vi "SentinelController v35 good v11.vi"() -> ()   [LabVIEW 2011] (continued)
                                tunnel: w568 -> [w597]
                                shift-right: [w590] -> w555
                                shift-left: 0 -> [w589]
                                shift-right: [w586] -> w556
                                shift-left: 0 -> [w584]
                                i -> [w587]
                                n2144 = Increment(x=w584) -> (x+1=w585:i32)
                                n2145 = Increment(x=w589) -> (x+1=w588:i32)
                                n2146 = Increment(x=w587) -> (x+1=w605:i32)
                                n2147 = String Subset(string=w597, offset (0)=w587, length (rest)=1 ("length (rest)")) -> (substring=w593:string)
                                n2148 = Multiply(x=3, y=w605) -> (x*y=w599:i32)
                                n2149 = Equal?(x=w593, y="1") -> (x = y?=w591:bool)
                                n2150 = Decrement(x=w599) -> (x-1=w598:i32)
                                n2151 = Select(t=w588, s=w591, f=w589) -> (s? t:f=w590:i32)
                                n2152 = Index Array(array=w606, index=w598) -> (element=w603:string)
                                n2153 = Decimal String To Number(string=w603, offset=0) -> (number=w601:i32)  [unwired: 1 in, 1 out]
                                n2154 = Equal?(x=w601, y=1) -> (x = y?=w594:bool)
                                n2155 = And(x=w594, y=w591) -> (x .and. y?=w595:bool)
                                n2156 = Select(t=w585, s=w595, f=w584) -> (s? t:f=w586:i32)
                                }
                                n2157 = case shown="True" w572 {
                                frame False {
                                }
                                frame True {
                                n2158 = One Button Dialog(message="Warning:\nH1 Parallelism Mismatch!\nEither allow this from the system configuration tab\nor change the parallelism on H2. This message will\ncontinue until the problem is corrected.") -> ()  [unwired: 1 in, 1 out]
                                }
                                }
                                n2159 = local read "H1 Device Count"() -> (w564:u32)
                                n2160 = local read "H1 Good Units"() -> (w565:u32)
                                n2161 = Add(x=w565, y=w556) -> (x+y=w566:u32)
                                n2162 = Add(x=w564, y=w555) -> (x+y=w563:u32)
                                n2163 = local write "H1 Good Units"(w566) -> ()
                                n2164 = local write "H1 Device Count"(w563) -> ()
                                }
                                frame #4 {
                                n2165 = local read "H1 Device Count"() -> (w612:u32)
                                n2166 = Divide(x=w608, y=w607) -> (x/y=w609:dbl)
                                n2167 = local read "H1 Good Units"() -> (w613:u32)
                                n2168 = Multiply(x=w609, y=100.0) -> (x*y=w611:dbl)
                                n2169 = Divide(x=w613, y=w612) -> (x/y=w616:dbl)
                                n2170 = local write "H1 cycle yield hid"(w611) -> ()
                                n2171 = Multiply(x=w616, y=100.0) -> (x*y=w614:dbl)
                                n2172 = local write "H1 lot yield mon"(w614) -> ()
                                }
                                frame #5 {
                                n2173 = local read "H1 online"() -> (w617:bool)
                                n2174 = local read "POWER"() -> (w618:bool)
                                n2175 = Compound Arithmetic op=AND(w617, w618) -> (w619:bool)
                                n2176 = case shown="True" w619 {
                                frame False {
                                n2177 = local write "MT99XX tester states H1 hid"(SC_MT99XX_tester_states."closing bus" ("SC virtual tester states")) -> ()
                                }
                                frame True {
                                n2178 = local write "MT99XX tester states H1 hid"(SC_MT99XX_tester_states."polling *SITES?" ("SC virtual tester states")) -> ()
                                }
                                }
                                }
                                }
                                }
                                frame "closing bus" {
                                n2179 = local read "GPIB bus 1 traffic"() -> (w626:string)
                                n2180 = local write "Exit SC tester H1 StMach hid"(TRUE ("Exit H1 state machine hid")) -> ()
                                n2181 = local read "VISA bus 1 resource name out hid"() -> (w630:refnum<visa-resource-name>)
                                n2182 = local read "VISA bus 1 error out hid"() -> (w629:errorcluster)
                                n2183 = Concatenate Strings(w626, "\r\n", "Bus 1: closing " ("string")) -> (w624:string)
                                n2184 = local write "GPIB bus 1 traffic"(w624) -> ()
                                n2185 = VISA Close(VISA resource name=w630, error in (no error)=w629) -> (error out=w628:errorcluster)
                                n2186 = Unbundle By Name(w628) -> ("status"=w627:bool)
                                n2187 = local write "VISA bus 1 close error"(w627) -> ()
                                }
                              }
                            }
                            frame #1 {
                              n2188 = local read "Slow for  Diagnostics"() -> (w631:bool)
                              n2189 = case shown="False" w631 {
                                frame False {
                                }
                                frame True {
                                n2190 = local read "GPIB wait time (ms)"() -> (w632:u32)
                                n2191 = Wait (ms)(milliseconds to wait=w632) -> ()  [unwired: 1 out]
                                }
                              }
                            }
                          }
                        }
                        frame "Seiko-Epson NS6040" {
                          n2192 = local write "NS6040 tester states H1 hid"(SC_NS6040_tester_states."initializing bus" ("NS6040 tester states H1 hid")) -> ()
                          n2193 = while {
                            stop <- w634 stop-if-true
                            n2194 = flat-sequence {
                              frame #0 {
                                n2195 = local read "NS6040 tester states H1 hid"() -> (w635:T4)
                                n2196 = case shown="\"testing\"" w635 {
                                frame "initializing bus", Default {
                                n2197 = flat-sequence {
                                frame #0 {
                                # "bus 1"
                                n2198 = local read "GPIB wait timeout hid"() -> (w639:u32)
                                n2199 = local read "SentCtrl talks to handler 1 at"() -> (w640:refnum<visa-resource-name>)
                                n2200 = local read "GPIB wait timeout hid"() -> (w638:u32)
                                n2201 = VISA Open(timeout (0)=w639, VISA resource name=w640) -> (VISA resource name=w637:refnum<visa-resource-name>, error out=w642:errorcluster)  [unwired: 3 in]
                                n2202 = property class="GPIB Instr"(reference=w637, error in=w642, "Timeout"=w638) -> (error out=w636:errorcluster)  [unwired: 1 out]
                                n2203 = local write "VISA bus 1 resource name out hid"(w637) -> ()
                                n2204 = Unbundle By Name(w636) -> ("status"=w641:bool)
                                n2205 = local write "VISA bus 1 open error"(w641) -> ()
                                n2206 = local write "VISA bus 1 error out hid"(w636) -> ()
                                }
                                frame #1 {
                                n2207 = local write "Exit SC tester H1 StMach hid"(FALSE ("Exit H1 state machine hid")) -> ()
                                n2208 = Concatenate Strings("Bus 1 initializing" ("string"), "\r\n") -> (w645:string)
                                n2209 = local write "GPIB bus 1 traffic"(w645) -> ()
                                }
                                frame #2 {
                                n2210 = local write "NS6040 tester states H1 hid"(SC_NS6040_tester_states."serial polling handler" ("NS6040 tester states H1 hid")) -> ()
                                }
                                }
                                }
                                frame "sending *IDN?" {
                                n2211 = flat-sequence {
                                tunnel: [w657] -> w650
                                tunnel: [w656] -> w649
                                tunnel: w650 -> [w671]
                                tunnel: w649 -> [w670]
                                tunnel: [w661] -> w648
                                tunnel: w648 -> [w672]
                                frame #0 {
                                w651 = "*IDN?\n"
                                # "It was discovered that his state is not initialized in application"
                                n2212 = local read "VISA bus 1 resource name out hid"() -> (w660:refnum<visa-resource-name>)
                                n2213 = local read "GPIB bus 1 traffic"() -> (w655:string)
                                n2214 = local read "VISA bus 1 error out hid"() -> (w659:errorcluster)
                                n2215 = Concatenate Strings(w655, "\r\n", "Bus 1 write: " ("string"), w651) -> (w653:string)
                                n2216 = VISA Write(VISA resource name=w660, write buffer=w651, error in (no error)=w659) -> (VISA resource name out=w657:refnum<visa-resource-name>, error out=w656:errorcluster)  [unwired: 1 out]
                                n2217 = Unbundle By Name(w656) -> ("status"=w658:bool)
                                n2218 = local write "GPIB bus 1 traffic"(w653) -> ()
                                n2219 = local write "GPIB bus 1 write error"(w658) -> ()
                                }
                                frame #1 {
                                n2220 = local read "GPIB bus 1 traffic"() -> (w663:string)
                                n2221 = VISA Read(VISA resource name=w671, byte count=u32 256, error in (no error)=w670) -> (VISA resource name out=w668:refnum<visa-resource-name>, read buffer=w662:string, error out=w667:errorcluster)  [unwired: 1 out]
                                n2222 = local write "VISA bus 1 resource name out hid"(w668) -> ()
                                n2223 = Unbundle By Name(w667) -> ("status"=w661:bool)
                                n2224 = local write "H1 response to *IDN? hid"(w662) -> ()
                                n2225 = local write "GPIB bus 1 read error"(w661) -> ()
                                n2226 = Concatenate Strings(w663, "\r\n", "Bus 1 read: " ("string"), w662) -> (w665:string)
                                n2227 = local write "GPIB bus 1 traffic"(w665) -> ()
                                }
                                frame #2 {
                                n2228 = case shown="False" w672 {
                                frame False {
                                n2229 = local write "NS6040 tester states H1 hid"(SC_NS6040_tester_states."serial polling handler" ("NS6040 tester states H1 hid")) -> ()
                                }
                                frame True {
                                n2230 = flat-sequence {
                                frame #0 {
                                n2231 = while {
                                stop <- w675 stop-if-true
                                n2232 = One Button Dialog(message="Warning:\nVirtual tester does not get a response\nto *IDN? from handler 1.\nCheck GPIB cable and that  handler 1 \nis running and ready to issue a start of test\nby responding with sites ready.", button name ("OK")="Dismiss and retry") -> (true=w675:bool)
                                n2233 = Wait (ms)(milliseconds to wait=u32 100) -> ()  [unwired: 1 out]
                                }
                                }
                                frame #1 {
                                n2234 = local write "H1 online"(FALSE ("H1 online")) -> ()
                                }
                                frame #2 {
                                n2235 = local write "NS6040 tester states H1 hid"(SC_NS6040_tester_states."sending *IDN?" ("NS6040 tester states H1 hid")) -> ()
                                }
                                }
                                }
                                }
                                }
                                }
                                }
                                frame "serial polling handler" {
                                w681 = "1"
                                w695 = "%08b"  # format string
                                n2236 = flat-sequence {
                                tunnel: [w716] -> w696
                                tunnel: [w715] -> _
                                frame #0 {
                                n2237 = local read "VISA bus 1 resource name out hid"() -> (w718:refnum<visa-resource-name>)
                                n2238 = local read "GPIB bus 1 traffic"() -> (w710:string)
                                n2239 = local read "VISA bus 1 error out hid"() -> (w717:errorcluster)
                                n2240 = VISA Read STB(8:w717, 11:w718) -> (0:w719:errorcluster, 2:w716:u16)  [unwired: 1 out]
                                n2241 = Concatenate Strings(w710, "\r\n", "Bus 1 read: " ("string"), "Serial polling handler 1") -> (w713:string)
                                n2242 = Unbundle By Name(w719) -> ("status"=w715:bool)
                                n2243 = local write "GPIB bus 1 traffic"(w713) -> ()
                                n2244 = local write "GPIB bus 1 write error"(w715) -> ()
                                }
                                }
                                n2245 = Format Into String "Format Into String"(format string=w695, w696) -> (resulting string=w682:string)  [unwired: 2 in, 1 out]
                                n2246 = local read "GPIB bus 1 traffic"() -> (w694:string)
                                n2247 = String Subset(string=w682, offset (0)=1, length (rest)=1 ("length (rest)")) -> (substring=w687:string)
                                n2248 = String Subset(string=w682, offset (0)=7, length (rest)=1 ("length (rest)")) -> (substring=w688:string)
                                n2249 = Equal?(x=w687, y=w681) -> (x = y?=w686:bool)
                                n2250 = Equal?(x=w681, y=w688) -> (x = y?=w685:bool)
                                n2251 = Concatenate Strings(w694, "\r\n", "Bus 1 read: " ("string"), w682) -> (w692:string)
                                n2252 = And(x=w686, y=w685) -> (x .and. y?=w680:bool)
                                n2253 = case shown="True" w680 {
                                frame False {
                                n2254 = flat-sequence {
                                frame #0 {
                                n2255 = Wait (ms)(milliseconds to wait=u32 1) -> ()  [unwired: 1 out]
                                }
                                frame #1 {
                                n2256 = local write "NS6040 tester states H1 hid"(SC_NS6040_tester_states."serial polling handler" ("NS6040 tester states H1 hid")) -> ()
                                }
                                }
                                }
                                frame True {
                                n2257 = flat-sequence {
                                frame #0 {
                                n2258 = local write "H1 Ready with sites"(TRUE ("H1 Ready with sites")) -> ()
                                }
                                frame #1 {
                                n2259 = Tick Count (ms)() -> (millisecond timer value=w700:u32)
                                n2260 = Tick Count (ms)() -> (millisecond timer value=w703:u32)
                                n2261 = local write "H1 wt start hidden"(w700) -> ()
                                n2262 = local write "H1 it end hidden"(w703) -> ()
                                n2263 = local write "H1 Indexing"(FALSE ("h1 indexing")) -> ()
                                n2264 = local write "H1 Testing"(FALSE ("h1 indexing")) -> ()
                                }
                                frame #2 {
                                n2265 = local read "H1 it start hidden"() -> (w707:u32)
                                n2266 = local read "H1 it end hidden"() -> (w708:u32)
                                n2267 = Subtract(x=w708, y=w707) -> (x-y=w704:u32)
                                n2268 = Divide(x=w704, y=u32 1000) -> (x/y=w706:dbl)
                                n2269 = local write "H1 measured Index Time"(w706) -> ()
                                }
                                frame #3 {
                                n2270 = local write "NS6040 tester states H1 hid"(SC_NS6040_tester_states."sending Fullsites?" ("NS6040 tester states H1 hid")) -> ()
                                }
                                }
                                }
                                }
                                n2271 = local write "GPIB bus 1 traffic"(w692) -> ()
                                }
                                frame "sending Fullsites?" {
                                n2272 = flat-sequence {
                                frame #0 {
                                n2273 = flat-sequence {
                                tunnel: [w727] -> w722
                                tunnel: [w726] -> w720
                                tunnel: [w732] -> w723
                                tunnel: w722 -> [w732]
                                tunnel: [w731] -> w721
                                tunnel: w720 -> [w731]
                                tunnel: w723 -> [w737]
                                tunnel: w721 -> [w736]
                                frame #0 {
                                w724 = "Fullsites?\n"
                                n2274 = local read "VISA bus 1 resource name out hid"() -> (w729:refnum<visa-resource-name>)
                                n2275 = local read "VISA bus 1 error out hid"() -> (w728:errorcluster)
                                n2276 = VISA Write(VISA resource name=w729, write buffer=w724, error in (no error)=w728) -> (VISA resource name out=w726:refnum<visa-resource-name>, error out=w727:errorcluster)  [unwired: 1 out]
                                n2277 = Unbundle By Name(w727) -> ("status"=w730:bool)
                                n2278 = call <vilib>:"Trim Whitespace.vi"("string"=w724) -> ("trimmed string"=w725:string)  [unwired: 1 in]
                                n2279 = local write "GPIB bus 1 write error"(w730) -> ()
                                n2280 = local write "GPIB bus 1 traffic"(w725) -> ()
                                }
                                frame #1 {
                                n2281 = Wait (ms)(milliseconds to wait=u32 2) -> ()  [unwired: 1 out]
                                }
                                frame #2 {
                                n2282 = local read "GPIB bus 1 traffic"() -> (w744:string)
                                n2283 = VISA Read(VISA resource name=w736, byte count=u32 256, error in (no error)=w737) -> (VISA resource name out=w739:refnum<visa-resource-name>, read buffer=w734:string, error out=w740:errorcluster)  [unwired: 1 out]
                                n2284 = local write "VISA bus 1 resource name out hid"(w739) -> ()
                                n2285 = local write "H1 FULLSITES? response hid"(w734) -> ()
                                n2286 = Unbundle By Name(w740) -> ("status"=w745:bool)
                                n2287 = local write "GPIB bus 1 read error"(w745) -> ()
                                n2288 = call <vilib>:"Trim Whitespace.vi"("string"=w734) -> ("trimmed string"=w735:string)  [unwired: 1 in]
                                n2289 = Concatenate Strings(w744, "\r\n", "Bus 1 read: " ("string"), w735) -> (w742:string)
                                n2290 = local write "GPIB bus 1 traffic"(w742) -> ()
                                }
                                }
                                }
                                frame #1 {
                                n2291 = local read "GPIB bus 1 read error"() -> (w746:bool)
                                n2292 = case shown="False" w746 {
                                frame False {
                                n2293 = flat-sequence {
                                frame #0 {
                                w755 = "%032b"  # format string
                                n2294 = local read "H1 FULLSITES? response hid"() -> (w748:string)
                                n2295 = call <vilib>:"Space Constant.vi"() -> ("String"=w750:string)
                                n2296 = Concatenate Strings("Fullsites" ("regular expression"), w750) -> (w749:string)
                                n2297 = call <vilib>:"Trim Whitespace.vi"("string"=w748) -> ("trimmed string"=w747:string)  [unwired: 1 in]
                                n2298 = Match Pattern(string=w747, regular expression=w749) -> (after substring=w753:string)  [unwired: 1 in, 3 out]
                                n2299 = Hexadecimal String To Number(string=w753, default (0uL)=u64 0 ("default (0 U32)")) -> (number=w756:u64)  [unwired: 1 in, 1 out]
                                n2300 = Format Into String "Format Into String"(format string=w755, w756) -> (resulting string=w752:string)  [unwired: 2 in, 1 out]
                                n2301 = local write "H1 FULLSITES? binary hid"(w752) -> ()
                                }
                                frame #1 {
                                n2302 = while {
                                stop <- w757 stop-if-true
                                n2303 = local read "H1 Lock"() -> (w757:bool)
                                n2304 = Wait (ms)(milliseconds to wait=u32 1) -> ()  [unwired: 1 out]
                                }
                                }
                                frame #2 {
                                n2305 = local write "NS6040 tester states H1 hid"(SC_NS6040_tester_states."testing" ("NS6040 tester states H1 hid")) -> ()
                                }
                                }
                                }
                                frame True {
                                n2306 = flat-sequence {
                                frame #0 {
                                n2307 = while {
                                stop <- w760 stop-if-true
                                n2308 = Wait (ms)(milliseconds to wait=u32 100) -> ()  [unwired: 1 out]
                                n2309 = One Button Dialog(message="Read error while reading FULLSITES?,\nclosing Bus and re-initializing" ("Reply from Sentinel Controller to tester")) -> (true=w760:bool)  [unwired: 1 in]
                                }
                                }
                                frame #1 {
                                n2310 = local read "VISA bus 1 resource name out hid"() -> (w766:refnum<visa-resource-name>)
                                n2311 = local read "VISA bus 1 error out hid"() -> (w765:errorcluster)
                                n2312 = VISA Close(VISA resource name=w766, error in (no error)=w765) -> (error out=w764:errorcluster)
                                n2313 = Unbundle By Name(w764) -> ("status"=w763:bool)
                                n2314 = local write "VISA bus 1 close error"(w763) -> ()
                                }
                                frame #2 {
                                n2315 = local write "VISA bus 1 close error"(FALSE ("H1 online")) -> ()
                                n2316 = local write "NS6040 tester states H1 hid"(SC_NS6040_tester_states."initializing bus" ("NS6040 tester states H1 hid")) -> ()
                                }
                                }
                                }
                                }
                                }
                                }
                                }
                                frame "testing" {
                                n2317 = flat-sequence {
                                frame #0 {
                                n2318 = local read "GPIB bus 1 traffic"() -> (w772:string)
                                n2319 = Concatenate Strings(w772, "\r\n", "Bus 1: " ("string"), "testing" ("string")) -> (w770:string)
                                n2320 = local write "GPIB bus 1 traffic"(w770) -> ()
                                }
                                frame #1 {
                                n2321 = Tick Count (ms)() -> (millisecond timer value=w777:u32)
                                n2322 = Tick Count (ms)() -> (millisecond timer value=w778:u32)
                                n2323 = local write "H1 Indexing"(FALSE ("waiting")) -> ()
                                n2324 = local write "H1 Testing"(TRUE ("testing")) -> ()
                                n2325 = local write "H1 Ready with sites"(FALSE ("H1 Ready with sites")) -> ()
                                n2326 = local write "H1 tt start hidden"(w777) -> ()
                                n2327 = local write "H1 wt end hidden"(w778) -> ()
                                }
                                frame #2 {
                                n2328 = local read "H1 wt start hidden"() -> (w782:u32)
                                n2329 = local read "H1 wt end hidden"() -> (w783:u32)
                                n2330 = Subtract(x=w783, y=w782) -> (x-y=w781:u32)
                                n2331 = Divide(x=w781, y=u32 1000) -> (x/y=w779:dbl)
                                n2332 = local write "H1 measured Wait Time"(w779) -> ()
                                }
                                frame #3 {
                                n2333 = while {
                                stop <- w785 continue-if-true
                                n2334 = local read "H1 Lock"() -> (w785:bool)
                                n2335 = Wait (ms)(milliseconds to wait=u32 1) -> ()  [unwired: 1 out]
                                }
                                }
                                frame #4 {
                                n2336 = local write "NS6040 tester states H1 hid"(SC_NS6040_tester_states."sending BINON?" ("NS6040 tester states H1 hid")) -> ()
                                }
                                }
                                }
                                frame "sending BINON?" {
                                n2337 = flat-sequence {
                                tunnel: [w800] -> w790
                                tunnel: [w799] -> w788
                                tunnel: w790 -> [w810]
                                tunnel: [w810] -> w789
                                tunnel: w788 -> [w809]
                                tunnel: [w809] -> w787
                                tunnel: w789 -> [w822]
                                tunnel: w787 -> [w821]
                                frame #0 {
                                n2338 = while {
                                i -> [w791]
                                stop <- w793 stop-if-true
                                n2339 = local read "Binning string from tester hid"() -> (w794:string)
                                n2340 = Wait (ms)(milliseconds to wait=u32 5) -> ()  [unwired: 1 out]
                                n2341 = String Length(string=w794) -> (length=w795:i32)
                                n2342 = Greater Than 0?(x=w795) -> (x > 0?=w793:bool)
                                "Numeric 2" <- w791
                                }
                                }
                                frame #1 {
                                n2343 = local write "H1 Ready with sites"(FALSE ("H1 Waiting")) -> ()
                                }
                                frame #2 {
                                # "2"
                                n2344 = local read "VISA bus 1 resource name out hid"() -> (w806:refnum<visa-resource-name>)
                                n2345 = local read "Binning string from tester hid"() -> (w797:string)
                                n2346 = local read "VISA bus 1 error out hid"() -> (w807:errorcluster)
                                n2347 = local read "GPIB bus 1 traffic"() -> (w804:string)
                                n2348 = VISA Write(VISA resource name=w806, write buffer=w797, error in (no error)=w807) -> (VISA resource name out=w799:refnum<visa-resource-name>, error out=w800:errorcluster)  [unwired: 1 out]
                                n2349 = local write "VISA bus 1 error out hid"(w800) -> ()
                                n2350 = Unbundle By Name(w800) -> ("status"=w805:bool)
                                n2351 = call <vilib>:"Trim Whitespace.vi"("string"=w797) -> ("trimmed string"=w798:string)  [unwired: 1 in]
                                n2352 = local write "GPIB bus 1 write error"(w805) -> ()
                                n2353 = Concatenate Strings(w804, "\r\n", "Bus 1 write: " ("string"), w798) -> (w802:string)
                                n2354 = local write "GPIB bus 1 traffic"(w802) -> ()
                                }
                                frame #3 {
                                n2355 = Wait (ms)(milliseconds to wait=u32 5) -> ()  [unwired: 1 out]
                                }
                                frame #4 {
                                # "3"
                                n2356 = local read "GPIB bus 1 traffic"() -> (w814:string)
                                n2357 = VISA Read(VISA resource name=w821, byte count=u32 256, error in (no error)=w822) -> (VISA resource name out=w819:refnum<visa-resource-name>, read buffer=w812:string, error out=w818:errorcluster)  [unwired: 1 out]
                                n2358 = local write "VISA bus 1 resource name out hid"(w819) -> ()
                                n2359 = Unbundle By Name(w818) -> ("status"=w813:bool)
                                n2360 = local write "GPIB bus 1 read error"(w813) -> ()
                                n2361 = call <vilib>:"Trim Whitespace.vi"("string"=w812) -> ("trimmed string"=w811:string)  [unwired: 1 in]
                                n2362 = Concatenate Strings(w814, "\r\n", "Bus 1 read: " ("string"), w811) -> (w816:string)
                                n2363 = local write "GPIB bus 1 traffic"(w816) -> ()
                                n2364 = local write "H1 echo hid"(w812) -> ()
                                }
                                frame #5 {
                                n2365 = while {
                                i -> [w823]
                                stop <- w824 continue-if-true
                                # "6"
                                n2366 = local read "Echo state of tester hid"() -> (w826:T3)
                                n2367 = Equal?(x=w826, y=Echo_tester_states."NO ECHO") -> (x = y?=w824:bool)
                                n2368 = Wait (ms)(milliseconds to wait=u32 5) -> ()  [unwired: 1 out]
                                "Numeric 3" <- w823
                                }
                                }
                                frame #6 {
                                n2369 = local read "GPIB bus 1 read error"() -> (w828:bool)
                                n2370 = case shown="False" w828 {
                                frame False {
                                n2371 = local read "Echo state of tester hid"() -> (w829:T3)
                                n2372 = case shown="\"ECHONG\", Default" w829 {
                                frame "ECHONG", Default {
                                n2373 = flat-sequence {
                                frame #0 {
                                n2374 = Wait (ms)(milliseconds to wait=u32 50) -> ()  [unwired: 1 out]
                                }
                                frame #1 {
                                n2375 = local write "NS6040 tester states H1 hid"(SC_NS6040_tester_states."sending ECHONG" ("NS6040 tester states H1 hid")) -> ()
                                }
                                }
                                }
                                frame "ECHOOK" {
                                n2376 = local write "NS6040 tester states H1 hid"(SC_NS6040_tester_states."sending ECHOOK" ("NS6040 tester states H1 hid")) -> ()
                                }
                                }
                                }
                                frame True {
                                n2377 = flat-sequence {
                                frame #0 {
                                n2378 = while {
                                stop <- w834 stop-if-true
                                n2379 = Wait (ms)(milliseconds to wait=u32 100) -> ()  [unwired: 1 out]
                                n2380 = One Button Dialog(message="Echo readback error for H1.\nClosing Bus 1.", button name ("OK")="Dismiss") -> (true=w834:bool)
                                }
                                }
                                frame #1 {
                                n2381 = local write "NS6040 tester states H1 hid"(SC_NS6040_tester_states."closing bus" ("NS6040 tester states H1 hid")) -> ()
                                }
                                }
                                }
                                }
                                }
                                }
                                }
                                frame "sending ECHONG" {
                                n2382 = flat-sequence {
                                frame #0 {
                                w838 = "ECHONG\n"
                                n2383 = local read "VISA bus 1 resource name out hid"() -> (w846:refnum<visa-resource-name>)
                                n2384 = local read "VISA bus 1 error out hid"() -> (w847:errorcluster)
                                n2385 = local read "GPIB bus 1 traffic"() -> (w844:string)
                                n2386 = VISA Write(VISA resource name=w846, write buffer=w838, error in (no error)=w847) -> (error out=w840:errorcluster)  [unwired: 2 out]
                                n2387 = Unbundle By Name(w840) -> ("status"=w845:bool)
                                n2388 = call <vilib>:"Trim Whitespace.vi"("string"=w838) -> ("trimmed string"=w839:string)  [unwired: 1 in]
                                n2389 = local write "VISA bus 1 error out hid"(w840) -> ()
                                n2390 = Concatenate Strings(w844, "\r\n", "Bus 1 write: " ("string"), w839) -> (w842:string)
                                n2391 = local write "GPIB bus 1 traffic"(w842) -> ()
                                n2392 = local write "GPIB bus 1 write error"(w845) -> ()
                                }
                                frame #1 {
                                n2393 = while {
                                stop <- w848 stop-if-true
                                n2394 = Wait (ms)(milliseconds to wait=u32 100) -> ()  [unwired: 1 out]
                                n2395 = One Button Dialog(message="ECHO from handler 1 did not match BINON'\nError message from \"sending ECHONG\" state\nBINON message will be resent.") -> (true=w848:bool)  [unwired: 1 in]
                                }
                                }
                                frame #2 {
                                n2396 = local write "NS6040 tester states H1 hid"(SC_NS6040_tester_states."sending BINON?" ("NS6040 tester states H1 hid")) -> ()
                                }
                                }
                                }
                                frame "sending ECHOOK" {
                                n2397 = flat-sequence {
                                frame #0 {
                                w852 = "ECHOOK\n"
                                n2398 = local read "VISA bus 1 resource name out hid"() -> (w860:refnum<visa-resource-name>)
                                n2399 = local read "VISA bus 1 error out hid"() -> (w861:errorcluster)
                                n2400 = local read "GPIB bus 1 traffic"() -> (w858:string)
                                n2401 = VISA Write(VISA resource name=w860, write buffer=w852, error in (no error)=w861) -> (error out=w854:errorcluster)  [unwired: 2 out]
                                n2402 = Unbundle By Name(w854) -> ("status"=w859:bool)
                                n2403 = call <vilib>:"Trim Whitespace.vi"("string"=w852) -> ("trimmed string"=w853:string)  [unwired: 1 in]
                                n2404 = local write "VISA bus 1 error out hid"(w854) -> ()
                                n2405 = Concatenate Strings(w858, "\r\n", "Bus 1 write: " ("string"), w853) -> (w856:string)
                                n2406 = local write "GPIB bus 1 traffic"(w856) -> ()
                                n2407 = local write "GPIB bus 1 write error"(w859) -> ()
                                }
                                frame #1 {
                                n2408 = Tick Count (ms)() -> (millisecond timer value=w863:u32)
                                n2409 = Tick Count (ms)() -> (millisecond timer value=w864:u32)
                                n2410 = local write "H1 Ready with sites"(FALSE ("waiting")) -> ()
                                n2411 = local write "H1 Testing"(FALSE ("waiting")) -> ()
                                n2412 = local write "H1 Indexing"(TRUE ("waiting")) -> ()
                                n2413 = local write "H1 tt end hidden"(w863) -> ()
                                n2414 = local write "H1 it start hidden"(w864) -> ()
                                }
                                frame #2 {
                                n2415 = local read "H1 tt start hidden"() -> (w870:u32)
                                n2416 = local read "H1 tt end hidden"() -> (w871:u32)
                                n2417 = Subtract(x=w871, y=w870) -> (x-y=w869:u32)
                                n2418 = Divide(x=w869, y=u32 1000) -> (x/y=w867:dbl)
                                n2419 = local write "H1 measured Test Time"(w867) -> ()
                                }
                                frame #3 {
                                n2420 = local read "H1 binning string hid"() -> (w872:string)
                                n2421 = local read "H1 FULLSITES? binary hid"() -> (w888:string)
                                n2422 = String Subset(string=w872, offset (0)=6, length (rest)=35 ("length (rest)")) -> (substring=w884:string)
                                n2423 = local read "H1 Device Count"() -> (w873:u32)
                                n2424 = local read "H1 Good Units"() -> (w874:u32)
                                n2425 = Search and Replace String(replace all?=TRUE ("replace all? (F)"), input string=w884, search string=",") -> (result string=w878:string)  [unwired: 5 in, 3 out]
                                n2426 = Search and Replace String(replace all?=TRUE ("replace all? (F)"), input string=w888, search string="1") -> (number of replacements=w890:i32)  [unwired: 5 in, 3 out]
                                n2427 = Divide(x=w874, y=w873) -> (x/y=w877:dbl)
                                n2428 = Add(x=w890, y=w873) -> (x+y=w889:u32)
                                n2429 = Search and Replace String(replace all?=TRUE ("replace all? (F)"), input string=w878, search string="1") -> (number of replacements=w879:i32)  [unwired: 5 in, 3 out]
                                n2430 = local write "H1 Device Count"(w889) -> ()
                                n2431 = Add(x=w879, y=w874) -> (x+y=w887:u32)
                                n2432 = Multiply(x=w877, y=100.0) -> (x*y=w875:dbl)
                                n2433 = local write "H1 Good Units"(w887) -> ()
                                n2434 = local write "H1 cycle yield hid"(w875) -> ()
                                }
                                frame #4 {
                                n2435 = local read "H1 Device Count"() -> (w893:u32)
                                n2436 = local read "H1 Good Units"() -> (w894:u32)
                                n2437 = Divide(x=w894, y=w893) -> (x/y=w897:dbl)
                                n2438 = Multiply(x=w897, y=100.0) -> (x*y=w895:dbl)
                                n2439 = local write "H1 lot yield mon"(w895) -> ()
                                }
                                frame #5 {
                                n2440 = local read "H1 online"() -> (w900:bool)
                                n2441 = local read "POWER"() -> (w899:bool)
                                n2442 = Compound Arithmetic op=AND(w900, w899) -> (w898:bool)
                                n2443 = case shown="True" w898 {
                                frame False {
                                n2444 = local write "NS6040 tester states H1 hid"(SC_NS6040_tester_states."closing bus" ("NS6040 tester states H1 hid")) -> ()
                                }
                                frame True {
                                n2445 = local write "NS6040 tester states H1 hid"(SC_NS6040_tester_states."serial polling handler" ("NS6040 tester states H1 hid")) -> ()
                                }
                                }
                                }
                                }
                                }
                                frame "closing bus" {
                                n2446 = local read "GPIB bus 1 traffic"() -> (w907:string)
                                n2447 = local write "Exit SC tester H1 StMach hid"(TRUE ("Exit H1 state machine hid")) -> ()
                                n2448 = local read "VISA bus 1 resource name out hid"() -> (w911:refnum<visa-resource-name>)
                                n2449 = local read "VISA bus 1 error out hid"() -> (w910:errorcluster)
                                n2450 = Concatenate Strings(w907, "\r\n", "Bus 1: closing " ("string")) -> (w905:string)
                                n2451 = local write "GPIB bus 1 traffic"(w905) -> ()
                                n2452 = VISA Close(VISA resource name=w911, error in (no error)=w910) -> (error out=w909:errorcluster)
                                n2453 = Unbundle By Name(w909) -> ("status"=w908:bool)
                                n2454 = local write "VISA bus 1 close error"(w908) -> ()
                                }
                                }
                              }
                              frame #1 {
                                n2455 = local read "Slow for  Diagnostics"() -> (w912:bool)
                                n2456 = case shown="False" w912 {
                                frame False {
                                }
                                frame True {
                                n2457 = local read "GPIB wait time (ms)"() -> (w913:u32)
                                n2458 = Wait (ms)(milliseconds to wait=w913) -> ()  [unwired: 1 out]
                                }
                                }
                              }
                            }
                            n2459 = local read "Exit SC tester H1 StMach hid"() -> (w634:bool)
                          }
                        }
                      }
                    }
                  }
                }
              }
              n2460 = local read "POWER"() -> (w360:bool)
            }
            n2461 = while {
              stop <- w1814 continue-if-true
              n2462 = local read "H2 online"() -> (w1815:bool)
              n2463 = case shown="True" w1815 {
                frame False {
                }
                frame True {
                  n2464 = flat-sequence {
                    frame #0 {
                      n2465 = local write "Exit SC tester H2 StMach hid"(FALSE ("Exit H2 state machine hid")) -> ()
                    }
                    frame #1 {
                      n2466 = local read "H2 handler type"() -> (w1817:T2)
                      n2467 = case shown="\"Seiko-Epson NS6040\"" w1817 {
                        frame "Multitest" {
                          n2468 = local write "MT99XX tester states H2 hid"(SC_MT99XX_tester_states."initializing bus" ("MT99XX tester states H2 hid")) -> ()
                          n2469 = flat-sequence {
                            frame #0 {
                              n2470 = local read "MT99XX tester states H2 hid"() -> (w1819:T5)
                              n2471 = case shown="\"binning\"" w1819 {
                                frame "initializing bus", Default {
                                n2472 = flat-sequence {
                                frame #0 {
                                # "bus 2"
                                n2473 = local read "GPIB wait timeout hid"() -> (w1822:u32)
                                n2474 = local read "SentCtrl talks to handler 2 at"() -> (w1824:refnum<visa-resource-name>)
                                n2475 = local read "GPIB wait timeout hid"() -> (w1823:u32)
                                n2476 = VISA Open(timeout (0)=w1822, VISA resource name=w1824) -> (VISA resource name=w1821:refnum<visa-resource-name>, error out=w1826:errorcluster)  [unwired: 3 in]
                                n2477 = property class="GPIB Instr"(reference=w1821, error in=w1826, "Timeout"=w1823) -> (error out=w1820:errorcluster)  [unwired: 1 out]
                                n2478 = local write "VISA bus 2 resource name out hid"(w1821) -> ()
                                n2479 = Unbundle By Name(w1820) -> ("status"=w1825:bool)
                                n2480 = local write "VISA bus 2 error out hid"(w1820) -> ()
                                n2481 = local write "VISA bus 2 open error"(w1825) -> ()
                                }
                                frame #1 {
                                n2482 = local write "Exit SC tester H2 StMach hid"(FALSE ("Exit H2 state machine hid")) -> ()
                                n2483 = Concatenate Strings("Bus 2 initializing" ("string"), "\r\n") -> (w1829:string)
                                n2484 = local write "GPIB bus 2 traffic"(w1829) -> ()
                                }
                                frame #2 {
                                n2485 = local write "MT99XX tester states H2 hid"(SC_MT99XX_tester_states."sending *IDN?" ("SC virtual tester states")) -> ()
                                }
                                }
                                }
                                frame "sending *IDN?" {
                                n2486 = flat-sequence {
                                tunnel: [w1841] -> w1834
                                tunnel: [w1840] -> w1833
                                tunnel: w1834 -> [w1855]
                                tunnel: w1833 -> [w1854]
                                tunnel: [w1845] -> w1832
                                tunnel: w1832 -> [w1856]
                                frame #0 {
                                w1835 = "*IDN?"
                                n2487 = local read "VISA bus 2 resource name out hid"() -> (w1844:refnum<visa-resource-name>)
                                n2488 = local read "GPIB bus 2 traffic"() -> (w1839:string)
                                n2489 = local read "VISA bus 2 error out hid"() -> (w1843:errorcluster)
                                n2490 = Concatenate Strings(w1839, "\r\n", "Bus 2 write: " ("string"), w1835) -> (w1837:string)
                                n2491 = VISA Write(VISA resource name=w1844, write buffer=w1835, error in (no error)=w1843) -> (VISA resource name out=w1841:refnum<visa-resource-name>, error out=w1840:errorcluster)  [unwired: 1 out]
                                n2492 = local write "GPIB bus 2 traffic"(w1837) -> ()
                                n2493 = Unbundle By Name(w1840) -> ("status"=w1842:bool)
                                n2494 = local write "GPIB bus 2 write error"(w1842) -> ()
                                }
                                frame #1 {
                                n2495 = local read "GPIB bus 2 traffic"() -> (w1847:string)
                                n2496 = VISA Read(VISA resource name=w1855, byte count=u32 256, error in (no error)=w1854) -> (VISA resource name out=w1852:refnum<visa-resource-name>, read buffer=w1846:string, error out=w1851:errorcluster)  [unwired: 1 out]
                                n2497 = local write "VISA bus 2 resource name out hid"(w1852) -> ()
                                n2498 = Unbundle By Name(w1851) -> ("status"=w1845:bool)
                                n2499 = local write "H2 response to *IDN? hid"(w1846) -> ()
                                n2500 = local write "GPIB bus 2 read error"(w1845) -> ()
                                n2501 = Concatenate Strings(w1847, "\r\n", "Bus 2 read: " ("string"), w1846) -> (w1849:string)
                                n2502 = local write "GPIB bus 2 traffic"(w1849) -> ()
                                }
                                frame #2 {
                                n2503 = case shown="False" w1856 {
                                frame False {
                                n2504 = local write "MT99XX tester states H2 hid"(SC_MT99XX_tester_states."polling *SITES?" ("SC virtual tester states")) -> ()
                                }
                                frame True {
                                n2505 = flat-sequence {
                                frame #0 {
                                n2506 = while {
                                stop <- w1859 stop-if-true
                                n2507 = One Button Dialog(message="Warning:\nVirtual tester does not get a response\nto *IDN? from handler 2.\nCheck GPIB cable and that  handler 2 \nis running and ready to issue a start of test\nby responding with sites ready.", button name ("OK")="Dismiss and retry") -> (true=w1859:bool)
                                n2508 = Wait (ms)(milliseconds to wait=u32 100) -> ()  [unwired: 1 out]
                                }
                                }
                                frame #1 {
                                n2509 = local write "H2 online"(FALSE ("H2 online")) -> ()
                                }
                                frame #2 {
                                n2510 = local write "MT99XX tester states H2 hid"(SC_MT99XX_tester_states."sending *IDN?" ("SC virtual tester states")) -> ()
                                }
                                }
                                }
                                }
                                }
                                }
                                }
                                frame "polling *SITES?" {
                                n2511 = flat-sequence {
                                tunnel: [w1867] -> w1865
                                tunnel: [w1866] -> w1864
                                tunnel: w1865 -> [w1903]
                                tunnel: w1864 -> [w1902]
                                frame #0 {
                                n2512 = while {
                                tunnel: [w1871] -> w1867
                                tunnel: [w1868] -> w1866
                                stop <- w1870 stop-if-true
                                n2513 = stacked-sequence {
                                tunnel: [w1883] -> w1873
                                tunnel: [w1882] -> w1872
                                frame #0 {
                                w1878 = "*SITES?"
                                n2514 = local read "VISA bus 2 resource name out hid"() -> (w1875:refnum<visa-resource-name>)
                                n2515 = local read "VISA bus 2 error out hid"() -> (w1874:errorcluster)
                                n2516 = Concatenate Strings("Handler 2 cycle start" ("string"), "\r\n", "Bus 2 write: " ("string"), w1878) -> (w1880:string)
                                n2517 = VISA Write(VISA resource name=w1875, write buffer=w1878, error in (no error)=w1874) -> (VISA resource name out=w1883:refnum<visa-resource-name>, error out=w1882:errorcluster)  [unwired: 1 out]
                                n2518 = Unbundle By Name(w1882) -> ("status"=w1876:bool)
                                n2519 = local write "GPIB bus 2 traffic"(w1880) -> ()
                                n2520 = local write "GPIB bus 2 write error"(w1876) -> ()
                                }
                                }
                                n2521 = Wait (ms)(milliseconds to wait=u32 1) -> ()  [unwired: 1 out]
                                n2522 = flat-sequence {
                                tunnel: w1873 -> [w1901]
                                tunnel: w1872 -> [w1900]
                                tunnel: [w1887] -> w1871
                                tunnel: [w1885] -> w1870
                                tunnel: [w1884] -> w1868
                                frame #0 {
                                n2523 = local read "GPIB bus 2 traffic"() -> (w1892:string)
                                n2524 = VISA Read(VISA resource name=w1901, byte count=u32 256, error in (no error)=w1900) -> (read buffer=w1887:string, error out=w1898:errorcluster)  [unwired: 2 out]
                                n2525 = Unbundle By Name(w1898) -> ("status"=w1884:bool)
                                n2526 = String Length(string=w1887) -> (length=w1889:i32)
                                n2527 = Scan Value(string=w1887, format string="%b", default (0 dbl)=u8 0) -> (value=w1891:u8)  [unwired: 1 out]
                                n2528 = Concatenate Strings(w1892, "\r\n", "Bus 2 read: " ("string"), w1887) -> (w1894:string)
                                n2529 = local write "GPIB bus 2 read error"(w1884) -> ()
                                n2530 = Greater Than 0?(x=w1889) -> (x > 0?=w1888:bool)
                                n2531 = Greater Than 0?(x=w1891) -> (x > 0?=w1890:bool)
                                n2532 = local write "GPIB bus 2 traffic"(w1894) -> ()
                                n2533 = And(x=w1888, y=w1890) -> (x .and. y?=w1886:bool)
                                n2534 = Or(x=w1886, y=w1884) -> (x .or. y?=w1885:bool)
                                }
                                }
                                }
                                }
                                frame #1 {
                                n2535 = case shown="False" w1902 {
                                tunnel: w1903 -> [w1904 _]
                                frame False {
                                n2536 = flat-sequence {
                                tunnel: w1904 -> [w1905]
                                frame #0 {
                                n2537 = local write "H2 SITES? response hid"(w1905) -> ()
                                n2538 = String Length(string=w1905) -> (length=w1906:i32)
                                n2539 = local write "H2 parallelism"(w1906) -> ()
                                }
                                frame #1 {
                                # "This block adds zeroes (sites not ready)\nto SITES READY from handlers when the\nhandler is running at a lower parallelism\nthan the test program, but has the same\npin mapping for the active sites in common."
                                n2540 = local read "Program Parallelism"() -> (w1908:u32)
                                n2541 = local read "H2 allow lower parallelism"() -> (w1909:bool)
                                n2542 = local read "H2 parallelism"() -> (w1907:u32)
                                n2543 = Less?(x=w1907, y=w1908) -> (x < y?=w1910:bool)
                                n2544 = And(x=w1910, y=w1909) -> (x .and. y?=w1911:bool)
                                n2545 = case shown="False" w1911 {
                                frame False {
                                n2546 = local read "Program Parallelism"() -> (w1914:u32)
                                n2547 = local read "H2 parallelism"() -> (w1912:u32)
                                n2548 = Greater?(x=w1912, y=w1914) -> (0:w1913:bool)
                                n2549 = case shown="True" w1913 {
                                frame False {
                                # "parallelisms must match if arriving here"
                                n2550 = local write "MT99XX tester states H2 hid"(SC_MT99XX_tester_states."testing" ("SC virtual tester states")) -> ()
                                }
                                frame True {
                                n2551 = local write "POWER"(FALSE ("POWER")) -> ()
                                n2552 = local write "MT99XX tester states H2 hid"(SC_MT99XX_tester_states."closing bus" ("SC virtual tester states")) -> ()
                                n2553 = One Button Dialog(message="Fatal error 301:\nTest program cannot support higher\nparallelism on handler 2.\nThe Sentinel Controller program is shutting down.\nPlease correct the mismatch and restart.") -> ()  [unwired: 1 in, 1 out]
                                }
                                }
                                }
                                frame True {
                                n2554 = local read "Program Parallelism"() -> (w1924:u32)
                                n2555 = local read "H2 parallelism"() -> (w1922:u32)
                                n2556 = local read "H2 SITES? response hid"() -> (w1920:string)
                                n2557 = local write "MT99XX tester states H2 hid"(SC_MT99XX_tester_states."testing" ("SC virtual tester states")) -> ()
                                n2558 = Subtract(x=w1924, y=w1922) -> (x-y=w1923:u32)
                                n2559 = for {
                                N: w1923 -> [_]
                                shift-right: [w1925] -> w1919
                                shift-left: w1920 -> [w1926]
                                n2560 = Concatenate Strings(w1926, "0" ("string")) -> (w1925:string)
                                }
                                n2561 = local write "H2 SITES? response hid"(w1919) -> ()
                                }
                                }
                                }
                                frame #2 {
                                n2562 = Tick Count (ms)() -> (millisecond timer value=w1932:u32)
                                n2563 = Tick Count (ms)() -> (millisecond timer value=w1931:u32)
                                n2564 = local write "H2 Ready with sites"(TRUE ("H2 Waiting")) -> ()
                                n2565 = local write "H2 Indexing"(FALSE ("h1 indexing")) -> ()
                                n2566 = local write "H2 Testing"(FALSE ("h1 indexing")) -> ()
                                n2567 = local write "H2 wt start hidden"(w1932) -> ()
                                n2568 = local write "H2 it end hidden"(w1931) -> ()
                                }
                                frame #3 {
                                n2569 = local read "H2 it start hidden"() -> (w1936:u32)
                                n2570 = local read "H2 it end hidden"() -> (w1937:u32)
                                n2571 = Subtract(x=w1937, y=w1936) -> (x-y=w1933:u32)
                                n2572 = local write "MT99XX tester states H2 hid"(SC_MT99XX_tester_states."testing" ("SC virtual tester states")) -> ()
                                n2573 = Divide(x=w1933, y=u32 1000) -> (x/y=w1935:dbl)
                                n2574 = local write "H2 measured  Index Time"(w1935) -> ()
                                }
                                }
                                }
                                frame True {
                                n2575 = flat-sequence {
